vi "FaultState.vi"(8 "error in (no error)":errorcluster, 11 "Actual Start [i]":i64) -> (0 "error out":errorcluster, 2 "Cluster":T1, 3 "Numeric":i64)   [LabVIEW 2018]
uses:
  Type_Def/Type_Def Actuator Controls.ctl
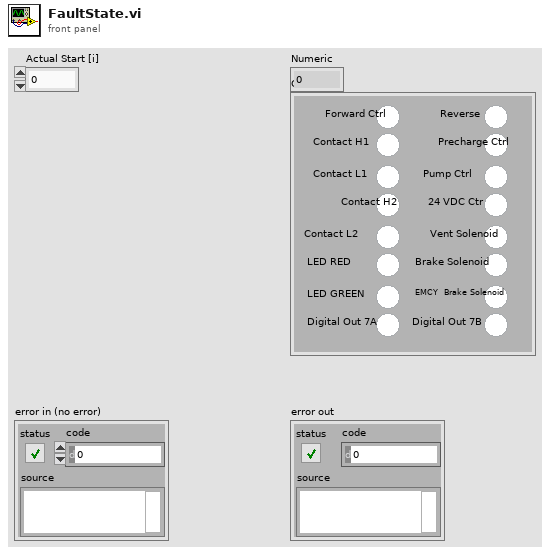
[diagram p1: front panel]
types:
  T1 = typedef "Type_Def Actuator Controls.ctl" = cluster{"Reverse ":bool, "Precharge Ctrl":bool, "Pump Ctrl":bool, "24 VDC Ctr":bool, "Vent Solenoid":bool, "Brake Solenoid":bool, "EMCY  Brake Solenoid":bool, "Digital Out 7B ":bool, "Forward Ctrl":bool, "Contact H1":bool, "Contact L1":bool, "Contact H2":bool, "Contact L2 ":bool, "LED RED":bool, "LED GREEN":bool, " Digital Out 7A":bool}
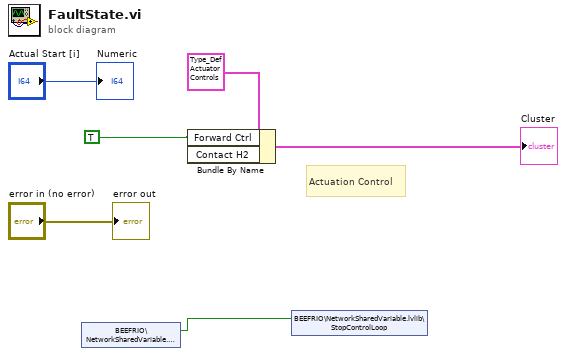
[diagram p0: block diagram]
diagram:
  w4 = TRUE
  # "Actuation Control"
  n1 = shared-variable "BEEFRIO\\NetworkSharedVariable.lvlib\\Shutdown"() -> (w1:bool)  [unwired: 1 in, 1 out]
  n2 = Bundle By Name(cluster=T1 {"Reverse "=FALSE, "Precharge Ctrl"=FALSE, "Pump Ctrl"=FALSE, "24 VDC Ctr"=FALSE, "Vent Solenoid"=FALSE, "Brake Solenoid"=FALSE, "EMCY  Brake Solenoid"=FALSE, "Digital Out 7B "=FALSE, "Forward Ctrl"=FALSE, "Contact H1"=FALSE, "Contact L1"=FALSE, "Contact H2"=FALSE, "Contact L2 "=FALSE, "LED RED"=FALSE, "LED GREEN"=FALSE, " Digital Out 7A"=FALSE} ("Cluster in 2"), "Forward Ctrl"=w4, "Contact H2"=w4) -> (→"Cluster":T1)
  n3 = shared-variable "BEEFRIO\\NetworkSharedVariable.lvlib\\StopControlLoop"(w1) -> ()  [unwired: 1 in, 1 out]
  "error out" <- "error in (no error)"
  "Numeric" <- "Actual Start [i]"
